vi "Get Device Info.vi"(8 "error in (no error)":errorcluster, 11 "image in":T1) -> (0 "error out":errorcluster, 3 "image out":T1)   [LabVIEW 2020, in "Point Grey Camera.lvclass"]
uses:
  Point Grey Camera.lvclass
  IMAQdx.ctl
  <resource>/objmgr/imaqdx.rc
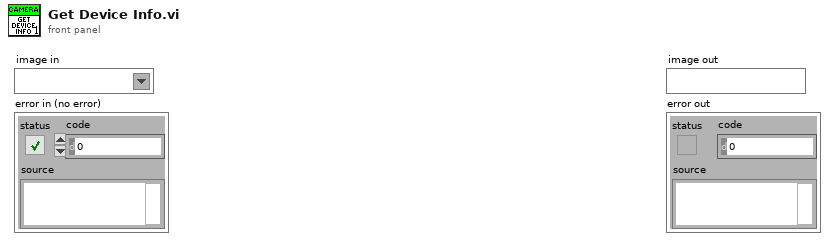
[diagram p1: front panel]
types:
  T1 = typedef "IMAQdx.ctl" = refnum<k21>
  T2 = typedef "mysql_authentication.ctl" = cluster{"User":string, "Password":string, "Database":string}
  T3 = cluster{"Port":u16, "IP Address":string, "Authentication":T2}
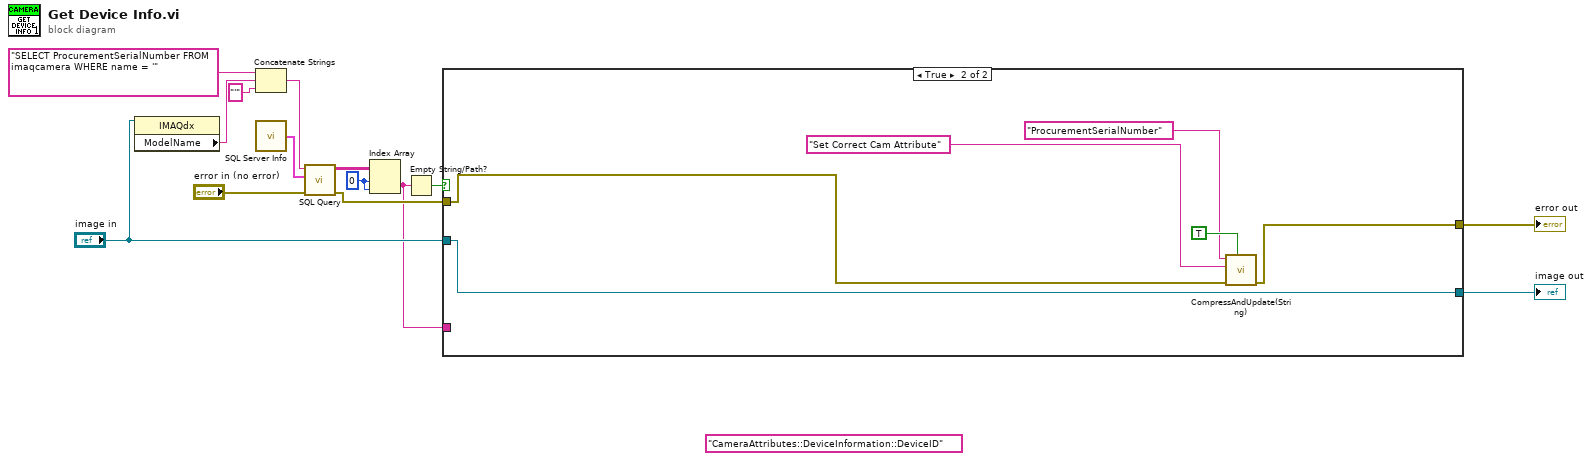
[diagram p0: block diagram]
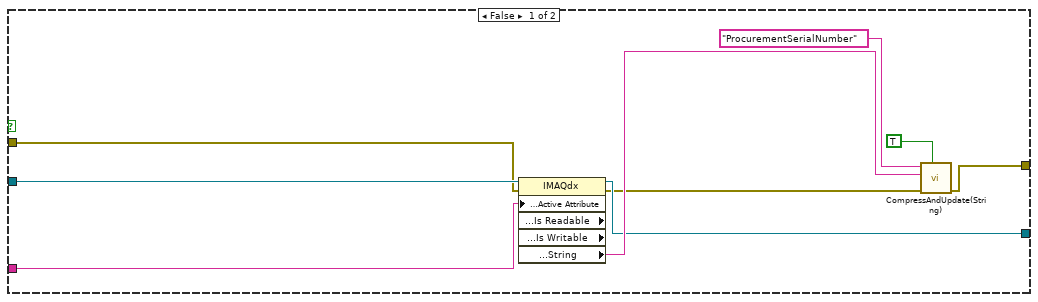
[diagram p2: hidden frame]
diagram:
  (unwired) "CameraAttributes::DeviceInformation::DeviceID" ("ActiveAttribute")
  w7 = 0 ("index (row)")
  n1 = property class="IMAQdx"(reference="image in") -> ("ModelName"=w11:string)  [unwired: 1 in, 2 out]
  n2 = Concatenate Strings("SELECT ProcurementSerialNumber FROM imaqcamera WHERE name = '" ("Query"), w11, "'" ("string")) -> (w10:string)
  n3 = call "SQL Server Info.vi"() -> ("SQL Server Info"=w9:T3)
  n4 = call "SQL Query.vi"("error in (no error)"="error in (no error)", "SQL Server Info"=w9, "Query"=w10) -> ("error out"=w4:errorcluster, "data"=w6:string[][])  [unwired: 7 in]
  n5 = Index Array(array=w6, index (row)=w7, index (col)=w7) -> (element=w3:string)
  n6 = Empty String/Path?(string/path=w3) -> (empty?=w5:bool)
  n7 = case shown="True" w5 {
    tunnel: "image in" -> [w20 w29]
    tunnel: w4 -> [w19 w25]
    tunnel: w3 -> [w18 _]
    tunnel: [w17 w29] -> w2
    tunnel: [w16 w26] -> w1
    frame False {
      n8 = property class="IMAQdx" props=["Camera Attributes:Active Attribute", "Camera Attributes:Is Readable", "Camera Attributes:Is Writable", "Camera Attributes:Value:String"](reference=w20, error in=w19, "Camera Attributes:Active Attribute"=w18) -> (reference out=w17:T1, error out=w15:errorcluster, "Camera Attributes:Value:String"=w21:string)  [unwired: 2 out]
      n9 = call "CompressAndUpdate(String).vi"("force CVT update (false)"=TRUE ("force CVT update"), "error in"=w15, "String"=w21, "command or variable name"="ProcurementSerialNumber") -> ("error out"=w16:errorcluster)  [unwired: 7 in]
    }
    frame True {
      n10 = call "CompressAndUpdate(String).vi"("force CVT update (false)"=TRUE ("force CVT update"), "error in"=w25, "String"="Set Correct Cam Attribute", "command or variable name"="ProcurementSerialNumber") -> ("error out"=w26:errorcluster)  [unwired: 7 in]
    }
  }
  "image out" <- w2
  "error out" <- w1
